vi "SingleApproach.vi"() -> ()   [LabVIEW 2014]
uses:
  <vilib>/rvi/Emulation/niFpgaGetClockAttributes.vi
  <vilib>/rvi/Emulation/niFpgaSctlEmulationGetInTimedLoop.vi
  <vilib>/rvi/Emulation/niFpgaEmulationReportErrorSimple.vi
  <vilib>/rvi/eio/common/nirviEmuTemplateMethod_errors.vi
  <vilib>/rvi/Emulation/niFpgaCriticalErrorInLSC.vi
  <vilib>/rvi/interface/RandomDataEmulation/niFpgaRandomDataHandleErrors.vi
  <vilib>/eio/EIONode/EIONode.xnode
  <vilib>/rvi/DataTransferAndStorage/Container/XNode/niFpgaContainer.xnode
  <vilib>/rvi/interface/RandomDataEmulation/nirviRandomDataFpgaReadWriteTemplate.vi
panel:
  in  "BaseCurrentRef":sgl
  out "PIZMaxPosIndex":i16
  in  "AppRate us":u32
  out "preCurrIndex":i16
  out "RealPosIndex":i16
  out "Approached?":bool
  out "PreCurrIndexDia":i16(graph)
  in  "stop":bool
  in  "Offset":i16
  out "PIZPosIndex":i16
  out "PIZPosIndexDia":i16(graph)
  out "Result":bool
  in  "Percentage %":sgl format="%#_13g"
  in  "BaseTime us":u32
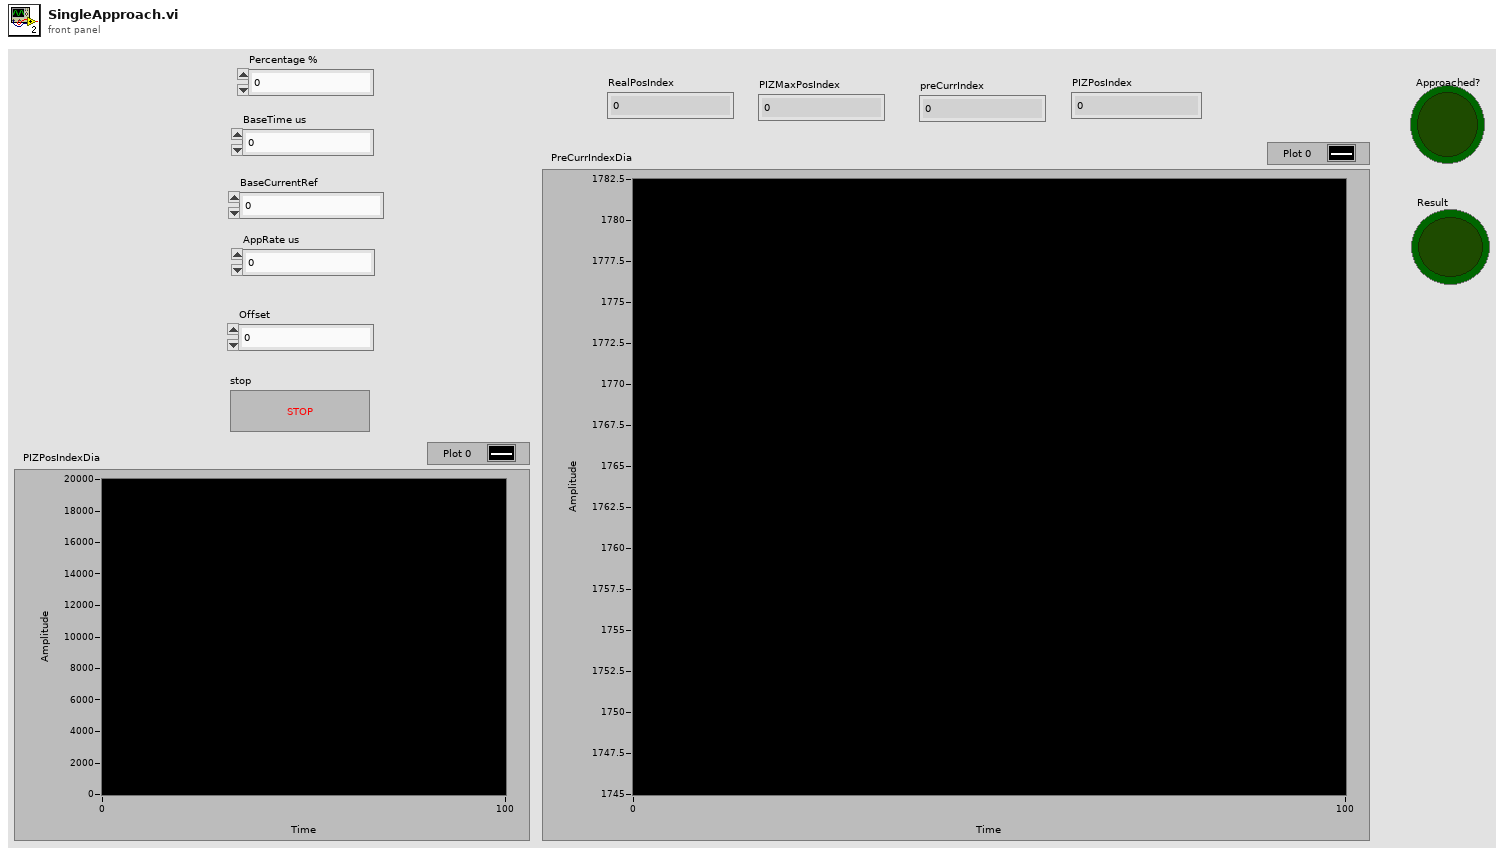
[diagram p1: front panel]
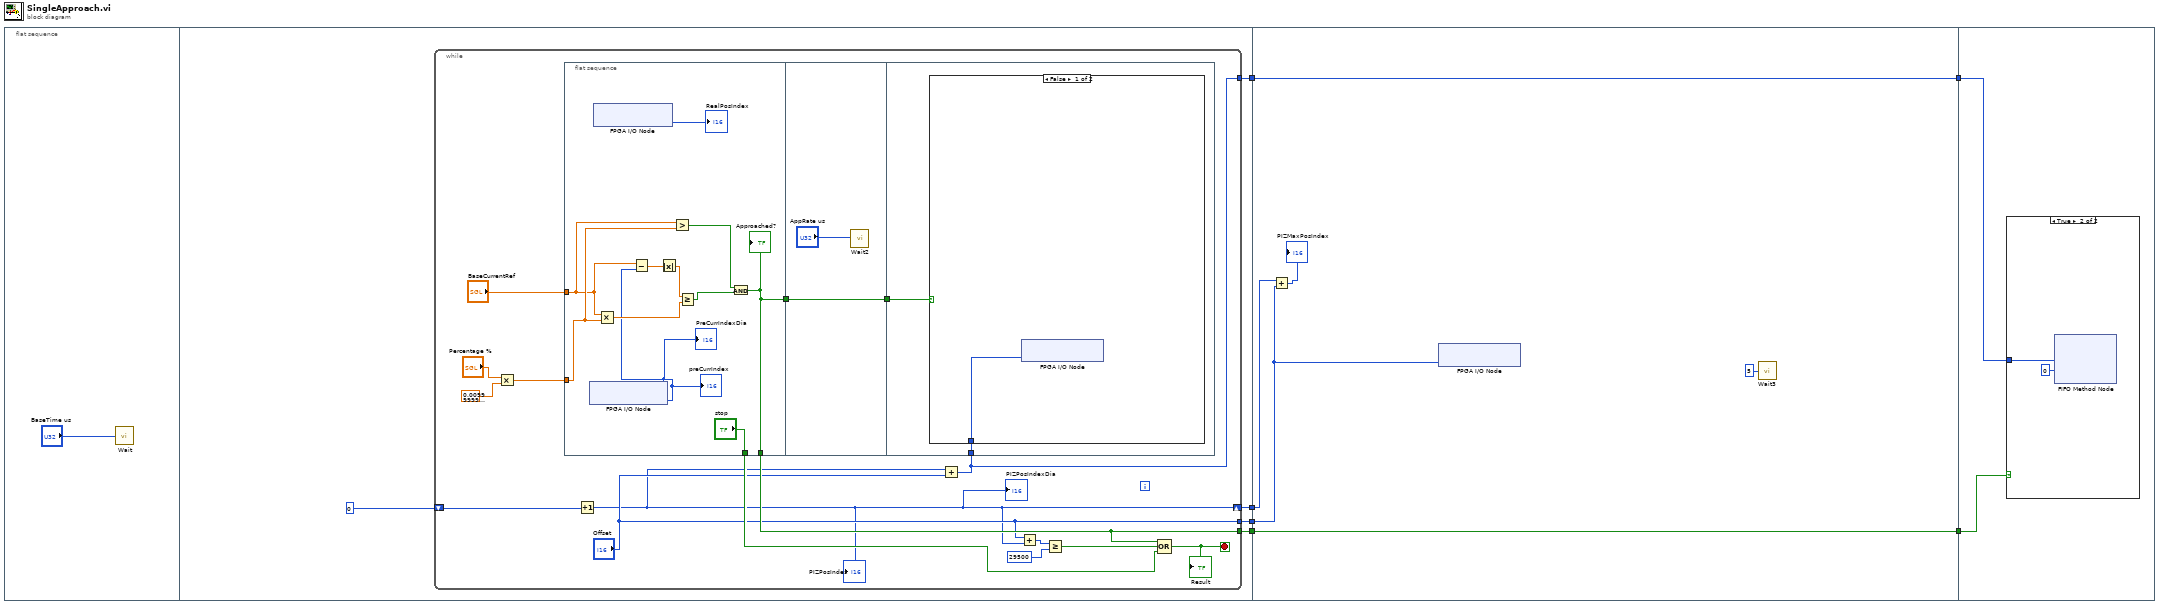
[diagram p0: block diagram]
diagram:
  n1 = flat-sequence {
    tunnel: [w11] -> w6
    tunnel: [w10] -> w5
    tunnel: [w9] -> w4
    tunnel: [w8] -> w3
    tunnel: w6 -> [w50]
    tunnel: w5 -> [w46]
    tunnel: w4 -> [w47]
    tunnel: [w50] -> w2
    tunnel: w3 -> [w49]
    tunnel: [w49] -> w1
    tunnel: w2 -> [w52]
    tunnel: w1 -> [w51]
    frame #0 {
      n2 = call "Wait"("Count(uSec)"="BaseTime us") -> ()  [unwired: 1 out]
    }
    frame #1 {
      n3 = while {
        shift-right: [w18] -> w9
        shift-left: i16 0 -> [w26]
        tunnel: [w25] -> w11
        tunnel: ["Offset"] -> w10
        tunnel: [w13] -> w8
        stop <- w22 stop-if-true
        n4 = Multiply(x="Percentage %", y=sgl 0.01) -> (x*y=w15:sgl)
        n5 = flat-sequence {
          tunnel: [w33] -> w28
          tunnel: [w33] -> w25
          tunnel: ["stop"] -> w21
          tunnel: w15 -> [w30]
          tunnel: "BaseCurrentRef" -> [w29]
          tunnel: w28 -> [w41]
          tunnel: [w41] -> w27
          tunnel: w27 -> [w43]
          tunnel: w13 -> [w42]
          frame #0 {
            n6 = xnode "FPGA I/O Node"() -> ("Connector0/AI1"=w35:i16)  [unwired: 1 in, 1 out]
            "preCurrIndex" <- w35
            "PreCurrIndexDia" <- w35
            n7 = xnode "FPGA I/O Node"() -> ("Connector0/AI0"=→"RealPosIndex":i16)  [unwired: 1 in, 1 out]
            n8 = Multiply(x=w29, y=w30) -> (x*y=w37:sgl)
            n9 = Subtract(x=w29, y=w35) -> (x-y=w39:sgl)
            n10 = Absolute Value(x=w39) -> (abs(x)=w38:sgl)
            n11 = Greater?(x=w29, y=w30) -> (0:w31:bool)
            n12 = Greater Or Equal?(x=w38, y=w37) -> (x >= y?=w32:bool)
            n13 = And(x=w31, y=w32) -> (x .and. y?=w33:bool)
            "Approached?" <- w33
          }
          frame #1 {
            n14 = call "Wait2"("Count(uSec)"="AppRate us") -> ()  [unwired: 1 out]
          }
          frame #2 {
            n15 = case shown="False" w43 {
              tunnel: w42 -> [w44 _]
              frame False {
                n16 = xnode "FPGA I/O Node"("Connector0/AO0"=w44) -> ()  [unwired: 1 in, 1 out]
              }
              frame True {
              }
            }
          }
        }
        n17 = Increment(x=w26) -> (x+1=w18:i16)
        "PIZPosIndex" <- w18
        "PIZPosIndexDia" <- w18
        n18 = Add(x=w18, y="Offset") -> (x+y=w13:i16)
        n19 = Add(x="Offset", y=w18) -> (x+y=w20:i16)
        n20 = Greater Or Equal?(x=w20, y=i16 29500) -> (x >= y?=w24:bool)
        n21 = Compound Arithmetic op=OR(w25, w24, w21) -> (w22:bool)
        "Result" <- w22
      }
    }
    frame #2 {
      n22 = Add(x=w47, y=w46) -> (x+y=→"PIZMaxPosIndex":i16)
      n23 = xnode "FPGA I/O Node"("Connector0/AO0"=w46) -> ()  [unwired: 1 in, 1 out]
      n24 = call "Wait3"("Count(uSec)"=u32 5) -> ()  [unwired: 1 out]
    }
    frame #3 {
      n25 = case shown="True" w52 {
        tunnel: w51 -> [_ w54]
        frame False {
        }
        frame True {
          n26 = xnode ("FIFO Method Node")("Element"=w54, "Timeout"=0) -> ()  [unwired: 1 in, 2 out]
        }
      }
    }
  }
